vi "Queue Image (iSUB) (SubVI).vi"(8 "Record":bool=TRUE, 10 "Image Size":T5={"Height"=512, "Width"=512}, 11 "Data Bundle":T1) -> (2 "Frame #":u32, 3 "Compression Ratio":dbl)   [LabVIEW 2015]
uses:
  Controls (HOST)/Image Size.ctl
  Controls (HOST)/Image Queue Bundle.ctl
  Controls (HOST)/REF.ctl
  Controls (HOST)/Data to Disk Bundle.ctl
  Controls (HOST)/FPGA REF (MWT).ctl
  Controls (HOST)/FPGA REF (iSUB).ctl
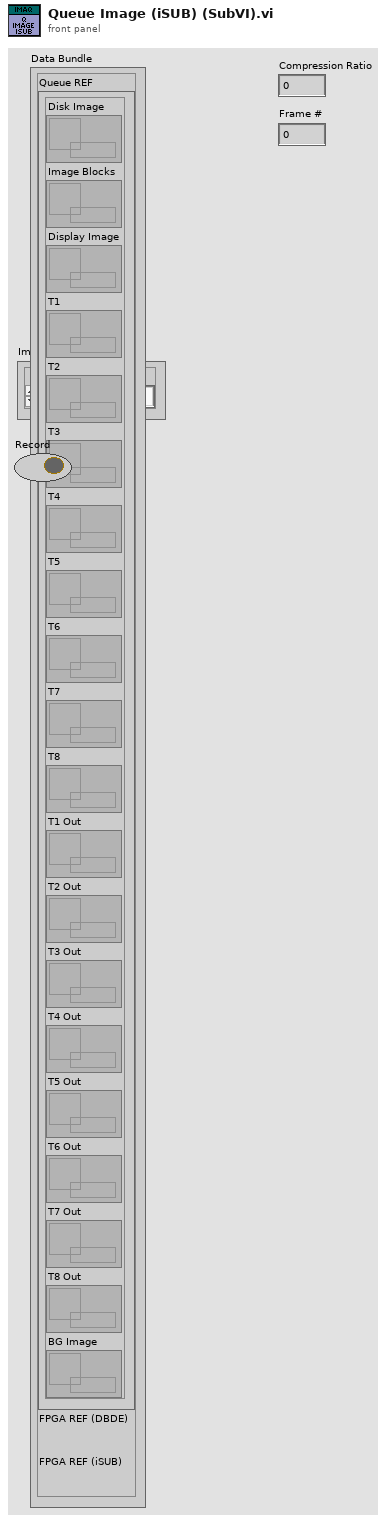
[diagram p1: front panel]
types:
  T1 = typedef "REF.ctl" = cluster{"Queue REF":T2, "FPGA REF (DBDE)":T3, "FPGA REF (iSUB)":T4}
  T2 = typedef "Image Queue Bundle.ctl" = cluster{"Disk Image":refnum<queue>, "Image Blocks":refnum<queue>, "Display Image":refnum<queue>, "T1":refnum<queue>, "T2":refnum<queue>, "T3":refnum<queue>, "T4":refnum<queue>, "T5":refnum<queue>, "T6":refnum<queue>, "T7":refnum<queue>, "T8":refnum<queue>, "T1 Out":refnum<queue>, "T2 Out":refnum<queue>, "T3 Out":refnum<queue>, "T4 Out":refnum<queue>, "T5 Out":refnum<queue>, "T6 Out":refnum<queue>, "T7 Out":refnum<queue>, "T8 Out":refnum<queue>, "BG Image":refnum<queue>}
  T3 = typedef "FPGA REF (MWT).ctl" = refnum<k20>
  T4 = typedef "FPGA REF (iSUB).ctl" = refnum<k20>
  T5 = typedef "Image Size.ctl" = cluster{"Height":u16, "Width":u16}
  T6 = typedef "Data to Disk Bundle.ctl" = cluster{"Frame Number":u64, "Time Stamp (x10ns)":u64, "Image Data":u64[], "Block Data":u64[], "Image REF":refnum<data-value>}
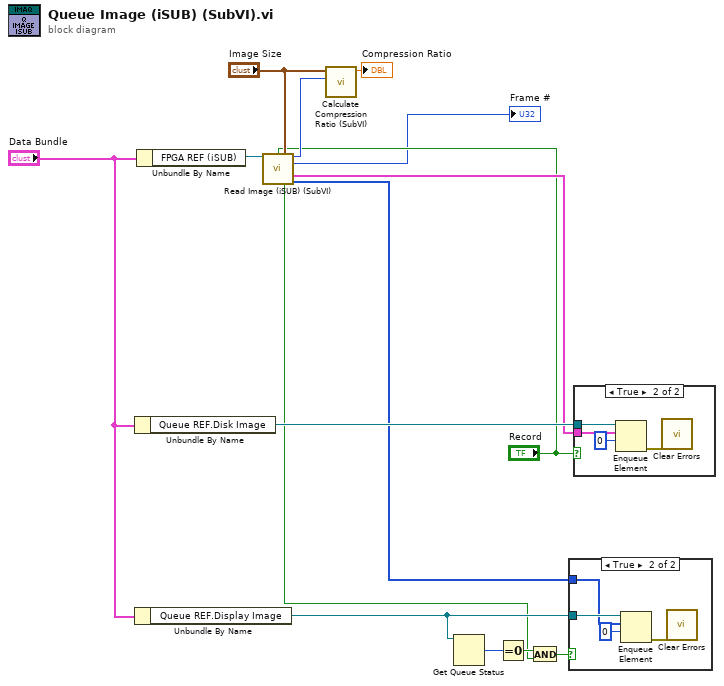
[diagram p0: block diagram]
diagram:
  n1 = Unbundle By Name("Data Bundle") -> ("Queue REF.Disk Image"=w15:refnum<queue>)
  n2 = Unbundle By Name("Data Bundle") -> ("Queue REF.Display Image"=w13:refnum<queue>)
  n3 = Unbundle By Name("Data Bundle") -> ("FPGA REF (iSUB)"=w4:T4)
  n4 = call "Read Image (iSUB) (SubVI).vi"("FPGA REF (iSUB)"=w4, "Send"="Record", "Image Size"="Image Size") -> ("N Compressed Bits"=w7:u32, "Frame #"=→"Frame #":u32, "Disk Data"=w5:T6, "Display?"=w3:bool, "Display Image"=w10:u64[])  [unwired: 8 in]
  n5 = call "Calculate Compression Ratio (SubVI).vi"("N Compressed Packets"=w7, "Image Size"="Image Size") -> ("Compression Ratio"=→"Compression Ratio":dbl)  [unwired: 9 in]
  n6 = Get Queue Status(queue=w13) -> (# elements in queue=w12:i32)  [unwired: 2 in, 7 out]
  n7 = Equal To 0?(x=w12) -> (x = 0?=w11:bool)
  n8 = And(x=w11, y=w3) -> (x .and. y?=w9:bool)
  n9 = case shown="True" w9 {
    tunnel: w13 -> [_ w19]
    tunnel: w10 -> [_ w16]
    frame False {
    }
    frame True {
      n10 = Enqueue Element(queue=w19, element=w16, timeout in ms (-1)=0) -> (error out=w18:errorcluster)  [unwired: 1 in, 2 out]
      n11 = call <vilib>:"Clear Errors.vi"("error in (no error)"=w18) -> ()  [unwired: 5 in, 2 out]
    }
  }
  n12 = case shown="True" "Record" {
    tunnel: w15 -> [_ w21]
    tunnel: w5 -> [_ w20]
    frame False {
    }
    frame True {
      n13 = Enqueue Element(queue=w21, element=w20, timeout in ms (-1)=0) -> (error out=w22:errorcluster)  [unwired: 1 in, 2 out]
      n14 = call <vilib>:"Clear Errors.vi"("error in (no error)"=w22) -> ()  [unwired: 5 in, 2 out]
    }
  }
